vi "Connect Paired Tunnels.vi"(8 "error in (no error)":errorcluster, 11 "CSM-Helper in":refnum<class "CSM-Helper.lvclass">) -> (0 "error out":errorcluster, 3 "CSM-Helper out":refnum<class "CSM-Helper.lvclass">)   [LabVIEW 2017, in "CSM-Helper.lvclass"]
doc: "### Connect Paired Tunnels.vi\n\n-- <b>Controls</b> --\n- <b>CSM-Helper in</b>: CSMHelper input\n\n-- <b>Indicators</b> --\n- <b>CSM-Helper out</b>: CSMHelper output"
uses:
  CSM-Helper.lvclass
  Utility/_Support/PairedTunnels.llb/csmHelper-PairedTunnels.lvlib
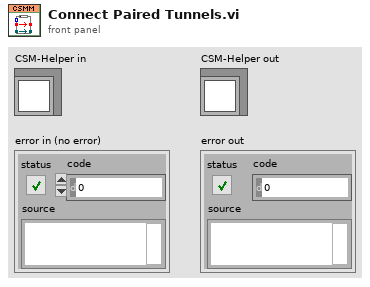
[diagram p1: front panel]
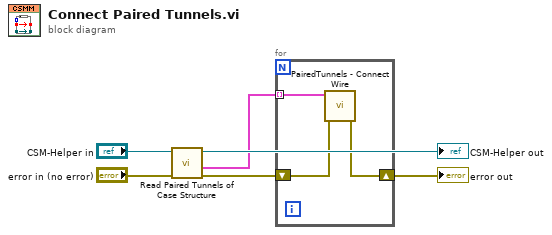
[diagram p0: block diagram]
diagram:
  n1 = call "Read Paired Tunnels of Case Structure.vi"("error in (no error)"="error in (no error)", "CSM-Helper in"="CSM-Helper in") -> ("error out"=w1:errorcluster, "Paired Tunnels"=w2:cluster{refnum<vi>, refnum<vi>}[], "CSM-Helper out"=→"CSM-Helper out":refnum<class "CSM-Helper.lvclass">)  [unwired: 7 in]
  n2 = for {
    tunnel: w2 -> [w9] mode=indexing
    shift-right: [w7] -> w3
    shift-left: w1 -> [w8]
    n3 = call "PairedTunnels - Connect Wire.vi"("Error in"=w8, "PairedTunnels"=w9) -> ("error out"=w7:errorcluster)  [unwired: 8 in, 1 out]
  }
  "error out" <- w3
